vi "get source path start.vi"(0 "main VI path":path) -> (4 "source file path":path)   [LabVIEW 2019]
doc: "This subVI uses the main VI's path as a reference pointer to choose the source data file path."
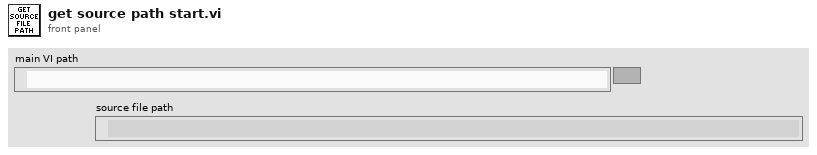
[diagram p1: front panel]
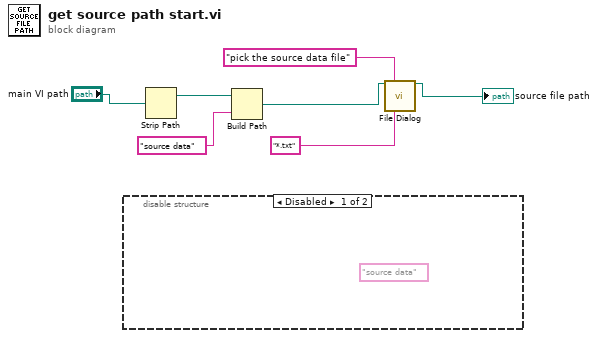
[diagram p0: block diagram]
diagram:
  n1 = disable-structure shown="Disabled" {
    frame Disabled {
      (unwired) "source data" ("default name")
    }
    frame Enabled {
    }
  }
  n2 = Strip Path(path="main VI path") -> (stripped path=w6:path)  [unwired: 1 out]
  n3 = Build Path(base path=w6, name or relative path="source data") -> (appended path=w3:path)
  n4 = call "File Dialog"("start path"=w3, "prompt"="pick the source data file", "pattern (all files)"="*.txt") -> ("selected path"=→"source file path":path)  [unwired: 9 in, 3 out]
